vi "GetPOVInput.vi"(1 "POV Input":dbl[](array[numeric])) -> (0 "POV Output":dbl[](array[numeric]))   [LabVIEW 2014]
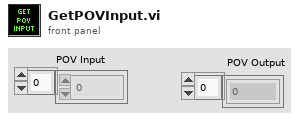
[diagram p1: front panel]
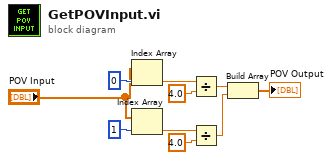
[diagram p0: block diagram]
diagram:
  n1 = Index Array(array="POV Input", index=0) -> (element=w2:dbl)
  n2 = Index Array(array="POV Input", index=1) -> (element=w1:dbl)
  n3 = Divide(x=w2, y=4.0) -> (x/y=w6:dbl)
  n4 = Divide(x=w1, y=4.0) -> (x/y=w5:dbl)
  n5 = Build Array(w6, w5) -> (→"POV Output":dbl[])
